vi "MenuHandler.vi"(5 "tree control":refnum<vi>, 7 "main queue":refnum<queue>, 8 "error in":errorcluster, 9 "parameters":variant, 10 "menu string":string, 11 "Abstract Engine":refnum<class "Abstract Engine.lvclass">) -> (0 "error out":errorcluster, 1 "refresh tree?":bool, 2 "Unhandled":bool, 3 "Abstract Engine out":refnum<class "Abstract Engine.lvclass">)   [LabVIEW 2025, in "Abstract Engine.lvlib" / "Abstract Engine.lvclass"]
doc: "Copyright 2017 National Instruments Corporation\n\nLicensed under the Apache License, Version 2.0 (the \"License\"); you may not use this file except in compliance with the License. You may obtain a copy of the License at http://www.apache.org/licenses/LICENSE-2.0\nUnless required by applicable law or agreed to in writing, software distributed under the License is distributed on an \"AS IS\" BASIS, WITHOUT WARRANTIES OR CONDITIONS OF ANY KIND, either express or implied. See the License for the specific language governing permissions and limitations under the License."
uses:
  Abstract Engine.lvclass
  Abstract Engine.lvclass/Abstract Engine.ctl
  Read Engine Cluster.vi
  Write Engine Cluster.vi
  Users/Public/Documents/Sandia National Labs/TSS Plugin/CEF.lvlibp/Node/ReadChildren.vi
  Users/Public/Documents/Sandia National Labs/TSS Plugin/CEF.lvlibp/Node/CEF_Node.lvclass
  Users/Public/Documents/Sandia National Labs/TSS Plugin/CEF.lvlibp/serializable node/CEF_serializable node.lvclass
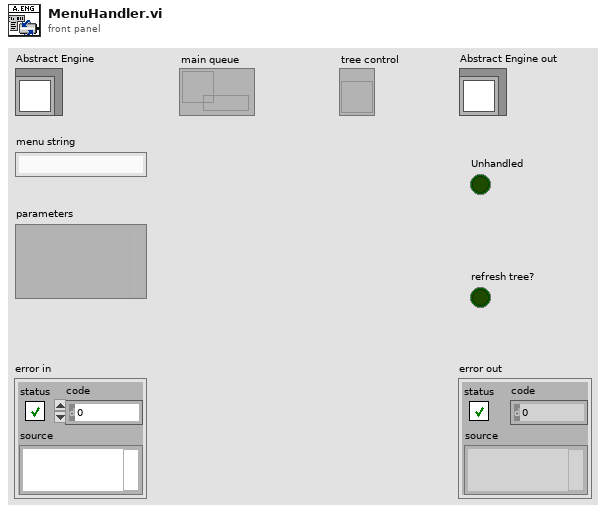
[diagram p1: front panel]
types:
  T1 = cluster{"notification":string, "Engine Data":string[]}
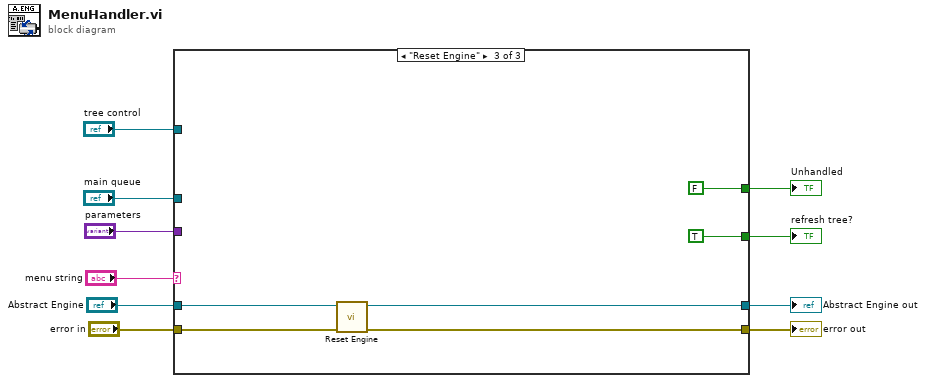
[diagram p0: block diagram]
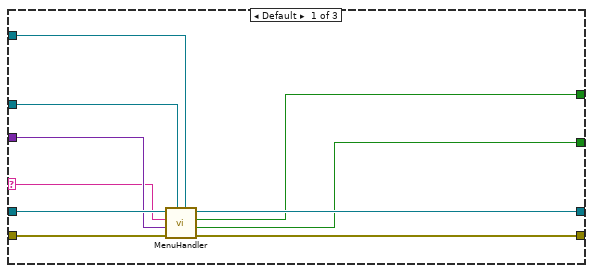
[diagram p2: hidden frame]
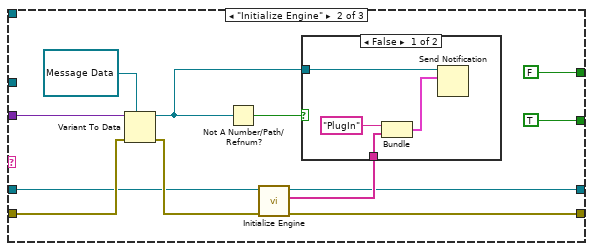
[diagram p3: hidden frame]
diagram:
  n1 = case shown="\"Reset Engine\"" "menu string" {
    selector: "menu string" -> [w15 _ _]
    tunnel: "Abstract Engine" -> [w18 w24 w42]
    tunnel: "error in" -> [w20 w28 w40]
    tunnel: [w19 w22 w39] -> w7
    tunnel: [w17 w21 w41] -> w6
    tunnel: [w12 FALSE ("Unhandled") FALSE ("Unhandled")] -> w5
    tunnel: [w11 TRUE ("refresh tree?") TRUE ("refresh tree?")] -> w4
    tunnel: "parameters" -> [w16 w30 _]
    tunnel: "main queue" -> [w14 _ _]
    tunnel: "tree control" -> [w13 _ _]
    frame Default {
      n2 = call-parent "MenuHandler.vi"("tree control"=w13, "main queue"=w14, "error in"=w20, "parameters"=w16, "menu string"=w15, "CEF_serializable node in"=w18) -> ("error out"=w19:errorcluster, "refresh tree?"=w11:bool, "Unhandled"=w12:bool, "CEF_serializable node out"=w17:refnum<class "Abstract Engine.lvclass">)  [unwired: 2 in]
    }
    frame "Initialize Engine" {
      n3 = Variant To Data(error in=w28, type=refnum<notifier> refnum ("notifier"), Variant=w30) -> (data=w26:refnum<notifier>, error out=w25:errorcluster)
      n4 = Not A Number/Path/Refnum?(number/path/refnum=w26) -> (NaN/Path/Refnum?=w27:bool)
      n5 = call "Initialize Engine.vi"("error in (no error)"=w25, "Abstract Engine"=w24) -> ("error out"=w22:errorcluster, "Engine Data"=w23:string[], "Abstract Engine out"=w21:refnum<class "Abstract Engine.lvclass">)  [unwired: 7 in]
      n6 = case shown="False" w27 {
        tunnel: w26 -> [w36 _]
        tunnel: w23 -> [w33 _]
        frame False {
          n7 = Bundle("notification"="PlugIn", "Engine Data"=w33) -> (w34:T1)  [unwired: 1 in]
          n8 = Send Notification(notification=w34, notifier=w36) -> ()  [unwired: 1 in, 2 out]
        }
        frame True {
        }
      }
    }
    frame "Reset Engine" {
      n9 = call "Reset Engine.vi"("error in (no error)"=w40, "Abstract Engine"=w42) -> ("error out"=w39:errorcluster, "Abstract Engine out"=w41:refnum<class "Abstract Engine.lvclass">)  [unwired: 8 in]
    }
  }
  "error out" <- w7
  "Abstract Engine out" <- w6
  "Unhandled" <- w5
  "refresh tree?" <- w4
